vi "FTW-JSON-Object-Update.vi"(0 "JSON Object":refnum<class "FTW-JSON.lvclass">, 5 "JSON Object to Merge":string, 7 "Update Mode":T1, 11 "error in":errorcluster) -> (4 "JSON Object out":refnum<class "FTW-JSON.lvclass">, 15 "error out":errorcluster)   [LabVIEW 2013, in "FTW-JSON.lvclass"]
uses:
  FTW-JSON.lvclass
  FTW-JSON-UpdateMode.ctl
  FTW-JSON.lvclass/FTW-JSON.ctl
panel:
  # "Inputs"
  # "Outputs"
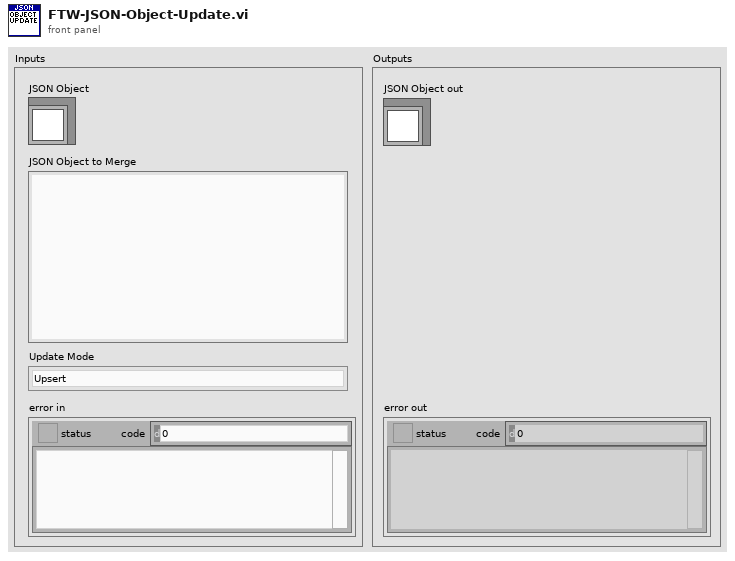
[diagram p1: front panel]
types:
  T1 = typedef "FTW-JSON.lvclass/FTW-JSON-UpdateMode.ctl" = enum16{"Upsert", "Update Only", "Insert Only"}
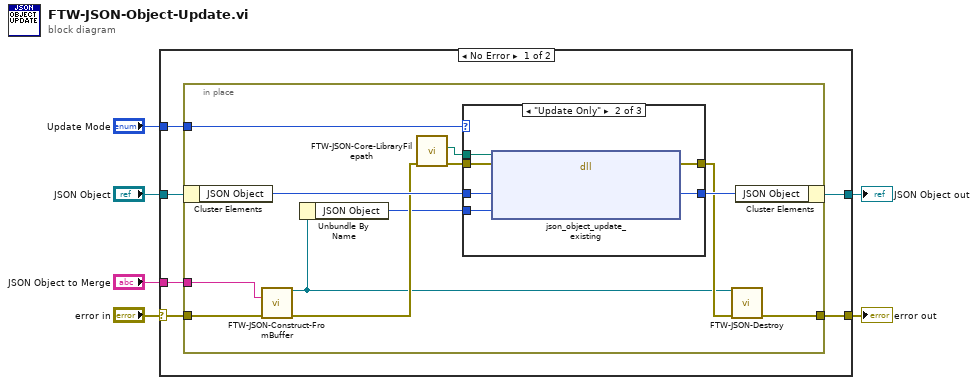
[diagram p0: block diagram]
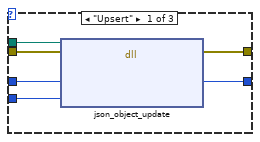
[diagram p2: hidden frame]
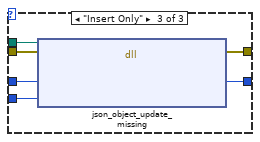
[diagram p3: hidden frame]
diagram:
  n1 = case shown="No Error" "error in" {
    selector: "error in" -> [w12 w44]
    tunnel: [w8 w44] -> w6
    tunnel: [w10 w43] -> w4
    tunnel: "JSON Object" -> [w11 w43]
    tunnel: "JSON Object to Merge" -> [w9 _]
    tunnel: "Update Mode" -> [w7 _]
    frame No Error {
      n2 = in-place {
        in-place-border: w12 -> [w19]
        in-place-border: w9 -> [w20]
        in-place-border: [w16] -> w8
        in-place-border: w7 -> [w13]
        n3 = in-place-cluster #1(w11) -> ("JSON Object"=w24:i64)
        n4 = call "FTW-JSON-Construct-FromBuffer.vi"("JSON String (UTF-8)"=w20, "error in"=w19) -> ("JSON Object"=w15:refnum<class "FTW-JSON.lvclass">, "error out"=w18:errorcluster)  [unwired: 12 in]
        n5 = Unbundle By Name(w15) -> ("JSON Object"=w14:i64)
        n6 = call "FTW-JSON-Core-LibraryFilepath.vi"("error in"=w18) -> ("error out"=w23:errorcluster, "JSON Library Filepath"=w22:path)  [unwired: 9 in]
        n7 = case shown="\"Update Only\"" w13 {
          tunnel: w24 -> [w30 w36 w42]
          tunnel: w23 -> [w29 w35 w41]
          tunnel: w22 -> [w28 w34 w40]
          tunnel: [w27 w33 w39] -> w21
          tunnel: [w26 w32 w38] -> w17
          tunnel: w14 -> [w25 w31 w37]
          frame "Upsert" {
            n8 = dll-call lib="?" fn="json_object_update"(path in=w28, error in=w29, "JSON Object ID"=w30, "JSON Object ID to Merge"=w25) -> (error out=w26:errorcluster, "JSON Object ID"=w27:i64)  [unwired: 3 in, 1 out]
          }
          frame "Update Only" {
            n9 = dll-call lib="?" fn="json_object_update_existing"(path in=w34, error in=w35, "JSON Object ID"=w36, "JSON Object ID to Merge"=w31) -> (error out=w32:errorcluster, "JSON Object ID"=w33:i64)  [unwired: 3 in, 1 out]
          }
          frame "Insert Only" {
            n10 = dll-call lib="?" fn="json_object_update_missing"(path in=w40, error in=w41, "JSON Object ID"=w42, "JSON Object ID to Merge"=w37) -> (error out=w38:errorcluster, "JSON Object ID"=w39:i64)  [unwired: 3 in, 1 out]
          }
        }
        n11 = call "FTW-JSON-Destroy.vi"("JSON Object"=w15, "error in"=w17) -> ("error out"=w16:errorcluster)  [unwired: 13 in]
        n12 = in-place-cluster #1("JSON Object"=w21) -> (w10:refnum<class "FTW-JSON.lvclass">)
      }
    }
    frame Error {
    }
  }
  "error out" <- w6
  "JSON Object out" <- w4
